vi "TJR_StateMachine.vi"() -> ()   [LabVIEW 2015]
uses:
  <vilib>/Utility/error.llb/DialogType.ctl
  <vilib>/DAQmx/read.llb/DAQmx Read (Analog 2D DBL NChan NSamp).vi
  <vilib>/DAQmx/configure/timing.llb/DAQmx Timing (Sample Clock).vi
  <vilib>/DAQmx/miscellaneous.llb/DAQmx Fill In Error Info.vi
  <vilib>/measure/maspectr.llb/Frequency Response Function (Mag-Phase) 1-1.vi
  <vilib>/express/express analysis/Spectral/Block/exnSpectralBlock spectral measurements RMS poly.vi
  <vilib>/express/express analysis/Spectral/Block/exnSpectralBlock spectral measurements RMS DDT.vi
  <vilib>/express/express analysis/Spectral/XNode/ExpressSpectralMeasurementsBlockNode.xnode
  <resource>/objmgr/daqmx.rc
  <vilib>/measure/NI_MAPro.lvlib
panel:
  in  "Tab Control":T1(tab)
  out "Measurement 8":dbl[](graph)
  out "Measurement 7":dbl[](graph)
  out "Measurement 6":dbl[](graph)
  out "Measurement 5":dbl[](graph)
  in  "Physical Channel 8":tag caption="Physical Channel"
  in  "Channel Name 8":string caption="Channel 8 Name"
  in  "Physical Channel 6":tag caption="Physical Channel"
  in  "Channel Name 6":string caption="Channel 6 Name"
  in  "Ch 8 On/Off":bool
  in  "Ch 6 On/Off":bool
  in  "Channel Type 8":u16(ring) caption="Channel Type" items=["Voltage", "Acceleration", "Current", "Other"]
  in  "Channel Type 7":u16(ring) caption="Channel Type" items=["Voltage", "Acceleration", "Current", "Other"]
  in  "Scale Factor 8":dbl[unit]=1.0
  in  "Scale Factor 6":dbl[unit]=1.0
  out "Ch 6 LED":bool
  out "Ch 8 LED":bool
  in  "Physical Channel 1":tag caption="Physical Channel"
  in  "Channel Name 1":string caption="Channel 1 Name"
  in  "Physical Channel 2":tag caption="Physical Channel"
  in  "Channel Name 2":string caption="Channel 2 Name"
  in  "Physical Channel 3":tag caption="Physical Channel"
  in  "Channel Name 3":string caption="Channel 3 Name"
  in  "Physical Channel 4":tag caption="Physical Channel"
  in  "Channel Name 4":string caption="Channel 4 Name"
  in  "Ch 1 On/Off":bool
  in  "Ch 2 On/Off":bool
  in  "Ch 3 On/Off":bool
  in  "Ch 4 On/Off":bool
  in  "Channel Type 1":u16(ring) caption="Channel Type" items=["Voltage", "Acceleration", "Current", "Other"]
  in  "Channel Type 3":u16(ring) caption="Channel Type" items=["Voltage", "Acceleration", "Current", "Other"]
  in  "Channel Type 4":u16(ring) caption="Channel Type" items=["Voltage", "Acceleration", "Current", "Other"]
  in  "Channel Type 2":u16(ring) caption="Channel Type" items=["Voltage", "Acceleration", "Current", "Other"]
  in  "Scale Factor 1":dbl[unit]=1.0 caption="mV/g"
  in  "Scale Factor 2":dbl[unit]=1.0 caption="mV/g"
  in  "Scale Factor 3":dbl[unit]=1.0 caption="mV/g"
  in  "Scale Factor 4":dbl[unit]=1.0
  in  "Rate":dbl=10.0 caption="Sampling Rate (Hz)" min=0.0 format="%0.2f"
  in  "Refresh Rate":dbl=5.0 caption="Refresh Rate (Hz)" min=1.0 max=20.0 step=1.0
  out "Measurement":dbl[](graph) caption="Input"
  out "Measurement 2":dbl[](graph) caption="A1"
  out "Measurement 3":dbl[](graph) caption="A2"
  out "Measurement 4":dbl[](graph) caption="A3"
  in  "Stop Acquisition":bool caption="stop"
  in  "Graph Time":dbl=10.0 caption="Graph Display Time (sec)" min=1.0 step=1.0
  out "Sampling Freq":dbl caption="Actual Sample Rate (Hz)"
  in  "Start Acquisition":bool
  in  "Exit":bool
  out "Ch 4 LED":bool
  out "Ch 3 LED":bool
  out "Ch 2 LED":bool
  out "Ch 1 LED":bool
  out "Ch 5 LED":bool
  in  "Scale Factor 5":dbl[unit]=1.0
  in  "Channel Type 6":u16(ring) caption="Channel Type" items=["Voltage", "Acceleration", "Current", "Other"]
  in  "Ch 5 On/Off":bool
  in  "Channel Name 5":string caption="Channel 5 Name"
  in  "Physical Channel 5":tag caption="Physical Channel"
  out "Ch 7 LED":bool
  in  "Scale Factor 7":dbl[unit]=1.0
  in  "Channel Type 5":u16(ring) caption="Channel Type" items=["Voltage", "Acceleration", "Current", "Other"]
  in  "Ch 7 On/Off":bool
  in  "Channel Name 7":string caption="Channel 7 Name"
  in  "Physical Channel 7":tag caption="Physical Channel"
  in  "Input Signal Measurement Channel":string(combo)
  out "A/O LED":bool
  out "Resulting Frequency":dbl=1000.0 format="%.4f"
  in  "Cycles per Buffer":i32=5 min=0 step=1
  in  "Waveform Type":T2(ring)
  in  "Amplitude":dbl=1.0 format="%.4f"
  in  "Analog Ouput On/Off":bool
  in  "Channel Name":string
  in  "Physical Channel":tag
  in  "Desired Frequency":dbl=100.0 min=0.0 format="%.4f"
  out "FFT Magnitude":dynamicdata(graph)
  out "FFT Phase":dynamicdata(graph)
  out "FRF Magnitude":cluster{"f0":dbl, "df":dbl, "magnitude":dbl[]}[](graph)
  out "FRF Phase":cluster{"f0":dbl, "df":dbl, "phase":dbl[]}[](graph)
  out "FRF Coherence":cluster{"f0":dbl, "df":dbl, "coherence":dbl[]}[](graph)
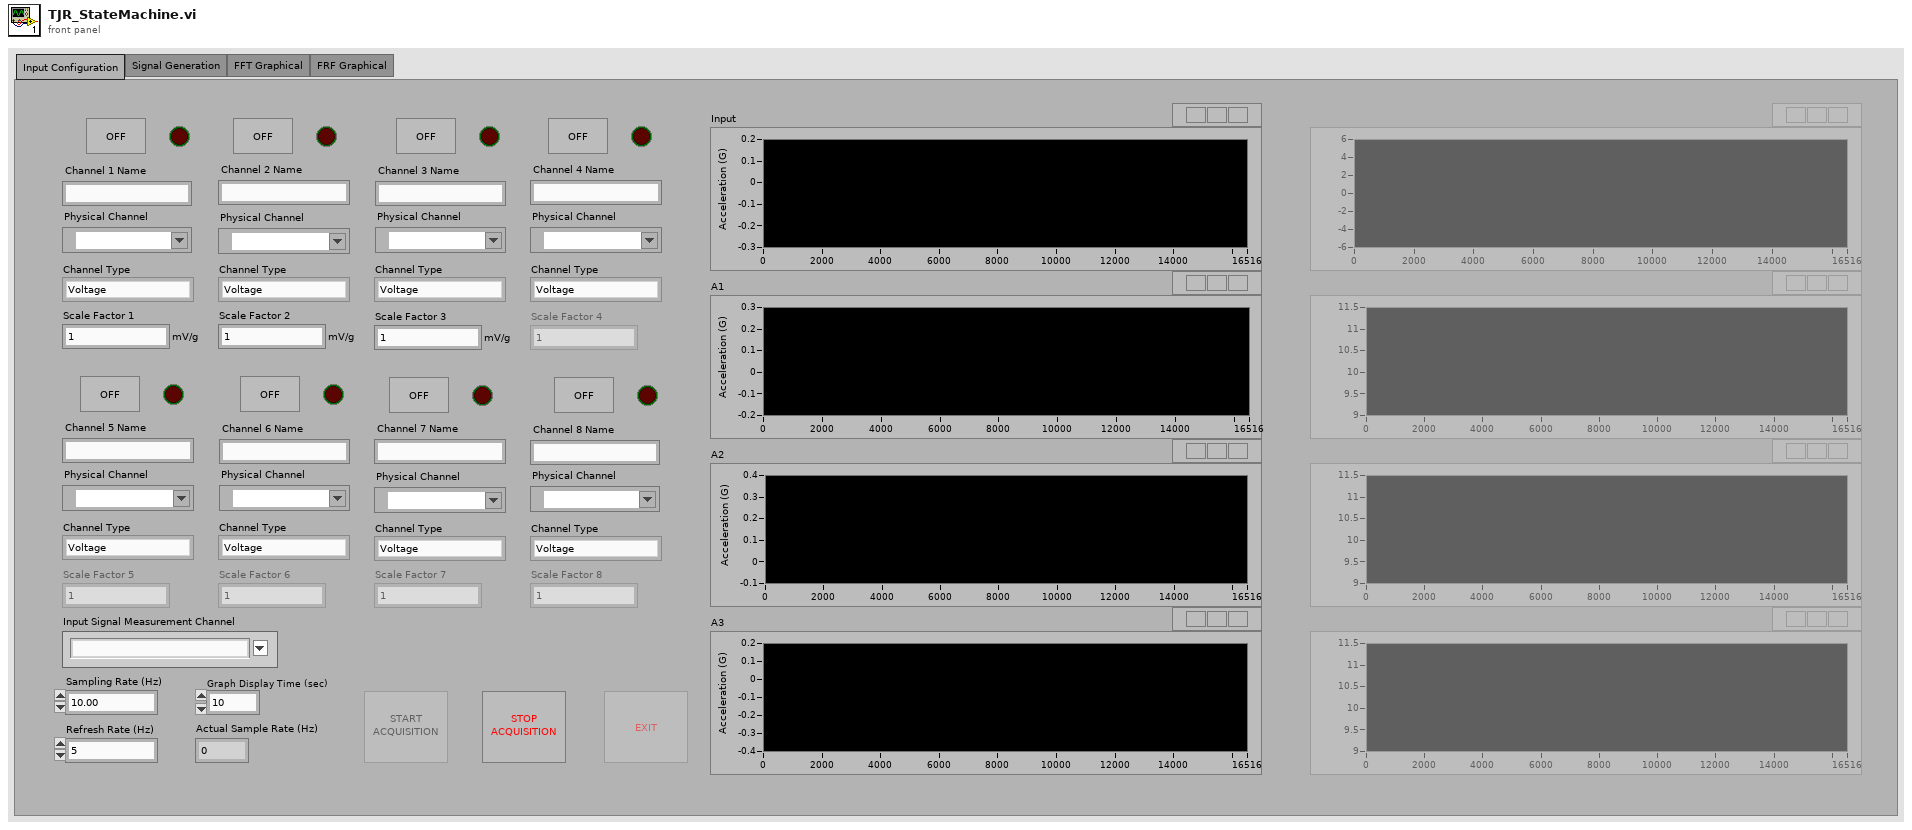
[diagram p1: front panel]
types:
  T1 = enum32{"Input Configuration", "Signal Generation", "FFT Graphical", "FRF Graphical"}
  T2 = enum16{"Sine Wave", "Triangle Wave", "Square Wave", "Sawtooth Wave"}
  T3 = cluster{"averaging mode":u16, "weighting mode":u16, "number of averages":u32}
  T4 = cluster{"dB On (F)":bool, "unwrap phase (F)":bool, "convert to degree (F)":bool}
  T5 = cluster{"Ch 1 On/Off":bool, "Ch 2 On/Off":bool, "Ch 3 On/Off":bool, "Ch 4 On/Off":bool, "Ch 5 On/Off":bool, "Ch 6 On/Off":bool, "Ch 7 On/Off":bool, "Ch 8 On/Off ":bool}
  T6 = cluster{"Physical Channel 1":tag, "Physical Channel 2":tag, "Physical Channel 3":tag, "Physical Channel 4":tag, "Physical Channel 5":tag, "Physical Channel 6":tag, "Physical Channel 7":tag, "Physical Channel 8":tag}
  T7 = cluster{"Minimum Value (V) 1":dbl, "Minimum Value (V) 2":dbl, "Minimum Value (V) 3":dbl, "Minimum Value (V) 4":dbl, "Minimum Value (V) 5":dbl, "Minimum Value (V) 6":dbl, "Minimum Value (V) 7":dbl, "Minimum Value (V) 8":dbl}
  T8 = cluster{"Scale Factor 8":dbl[unit], "Scale Factor 7":dbl[unit], "Scale Factor 6":dbl[unit], "Scale Factor 5":dbl[unit], "Scale Factor 4":dbl[unit], "Scale Factor 3":dbl[unit], "Scale Factor 2":dbl[unit], "Scale Factor 1":dbl[unit]}
  T9 = cluster{"Maximum Value (V) 1":dbl, "Maximum Value (V) 2":dbl, "Maximum Value (V) 3":dbl, "Maximum Value (V) 4":dbl, "Maximum Value (V) 5":dbl, "Maximum Value (V) 6":dbl, "Maximum Value (V) 7":dbl, "Maximum Value (V) 8":dbl}
  T10 = cluster{"Channel Name 1":string, "Channel Name 2":string, "Channel Name 3":string, "Channel Name 4":string, "Channel Name 5":string, "Channel Name 6":string, "Channel Name 7":string, "Channel Name 8":string}
  T11 = cluster{"Channel Type 1":u16, "Channel Type 2":u16, "Channel Type 3":u16, "Channel Type 4":u16, "Channel Type 5":u16, "Channel Type 6":u16, "Channel Type 7":u16, "Channel Type 8":u16}
  T12 = cluster{"Measurement":refnum<vi>, "Measurement 2":refnum<vi>, "Measurement 3":refnum<vi>, "Measurement 4":refnum<vi>, "Measurement 5":refnum<vi>, "Measurement 6":refnum<vi>, "Measurement 7":refnum<vi>, "Measurement 8":refnum<vi>}
  T13 = cluster{cluster{"Measurement":refnum<vi>, "Measurement 2":refnum<vi>, "Measurement 3":refnum<vi>, "Measurement 4":refnum<vi>, "Measurement 5":refnum<vi>, "Measurement 6":refnum<vi>, "Measurement 7":refnum<vi>, "Measurement 8":refnum<vi>}, cluster{"Ch 1 On/Off":bool, "Ch 2 On/Off":bool, "Ch 3 On/Off":bool, "Ch 4 On/Off":bool, "Ch 5 On/Off":bool, "Ch 6 On/Off":bool, "Ch 7 On/Off":bool, "Ch 8 On/Off ":bool}, cluster{"Channel Name 1":string, "Channel Name 2":string, "Channel Name 3":string, "Channel Name 4":string, "Channel Name 5":string, "Channel Name 6":string, "Channel Name 7":string, "Channel Name 8":string}, cluster{"Physical Channel 1":tag, "Physical Channel 2":tag, "Physical Channel 3":tag, "Physical Channel 4":tag, "Physical Channel 5":tag, "Physical Channel 6":tag, "Physical Channel 7":tag, "Physical Channel 8":tag}, cluster{"Maximum Value (V) 1":dbl, "Maximum Value (V) 2":dbl, "Maximum Value (V) 3":dbl, "Maximum Value (V) 4":dbl, "Maximum Value (V) 5":dbl, "Maximum Value (V) 6":dbl, "Maximum Value (V) 7":dbl, "Maximum Value (V) 8":dbl}, cluster{"Minimum Value (V) 1":dbl, "Minimum Value (V) 2":dbl, "Minimum Value (V) 3":dbl, "Minimum Value (V) 4":dbl, "Minimum Value (V) 5":dbl, "Minimum Value (V) 6":dbl, "Minimum Value (V) 7":dbl, "Minimum Value (V) 8":dbl}, cluster{"Channel Type 1":u16, "Channel Type 2":u16, "Channel Type 3":u16, "Channel Type 4":u16, "Channel Type 5":u16, "Channel Type 6":u16, "Channel Type 7":u16, "Channel Type 8":u16}, cluster{"Scale Factor 8":dbl[unit], "Scale Factor 7":dbl[unit], "Scale Factor 6":dbl[unit], "Scale Factor 5":dbl[unit], "Scale Factor 4":dbl[unit], "Scale Factor 3":dbl[unit], "Scale Factor 2":dbl[unit], "Scale Factor 1":dbl[unit]}}
  T14 = typedef "DialogType.ctl" = u16
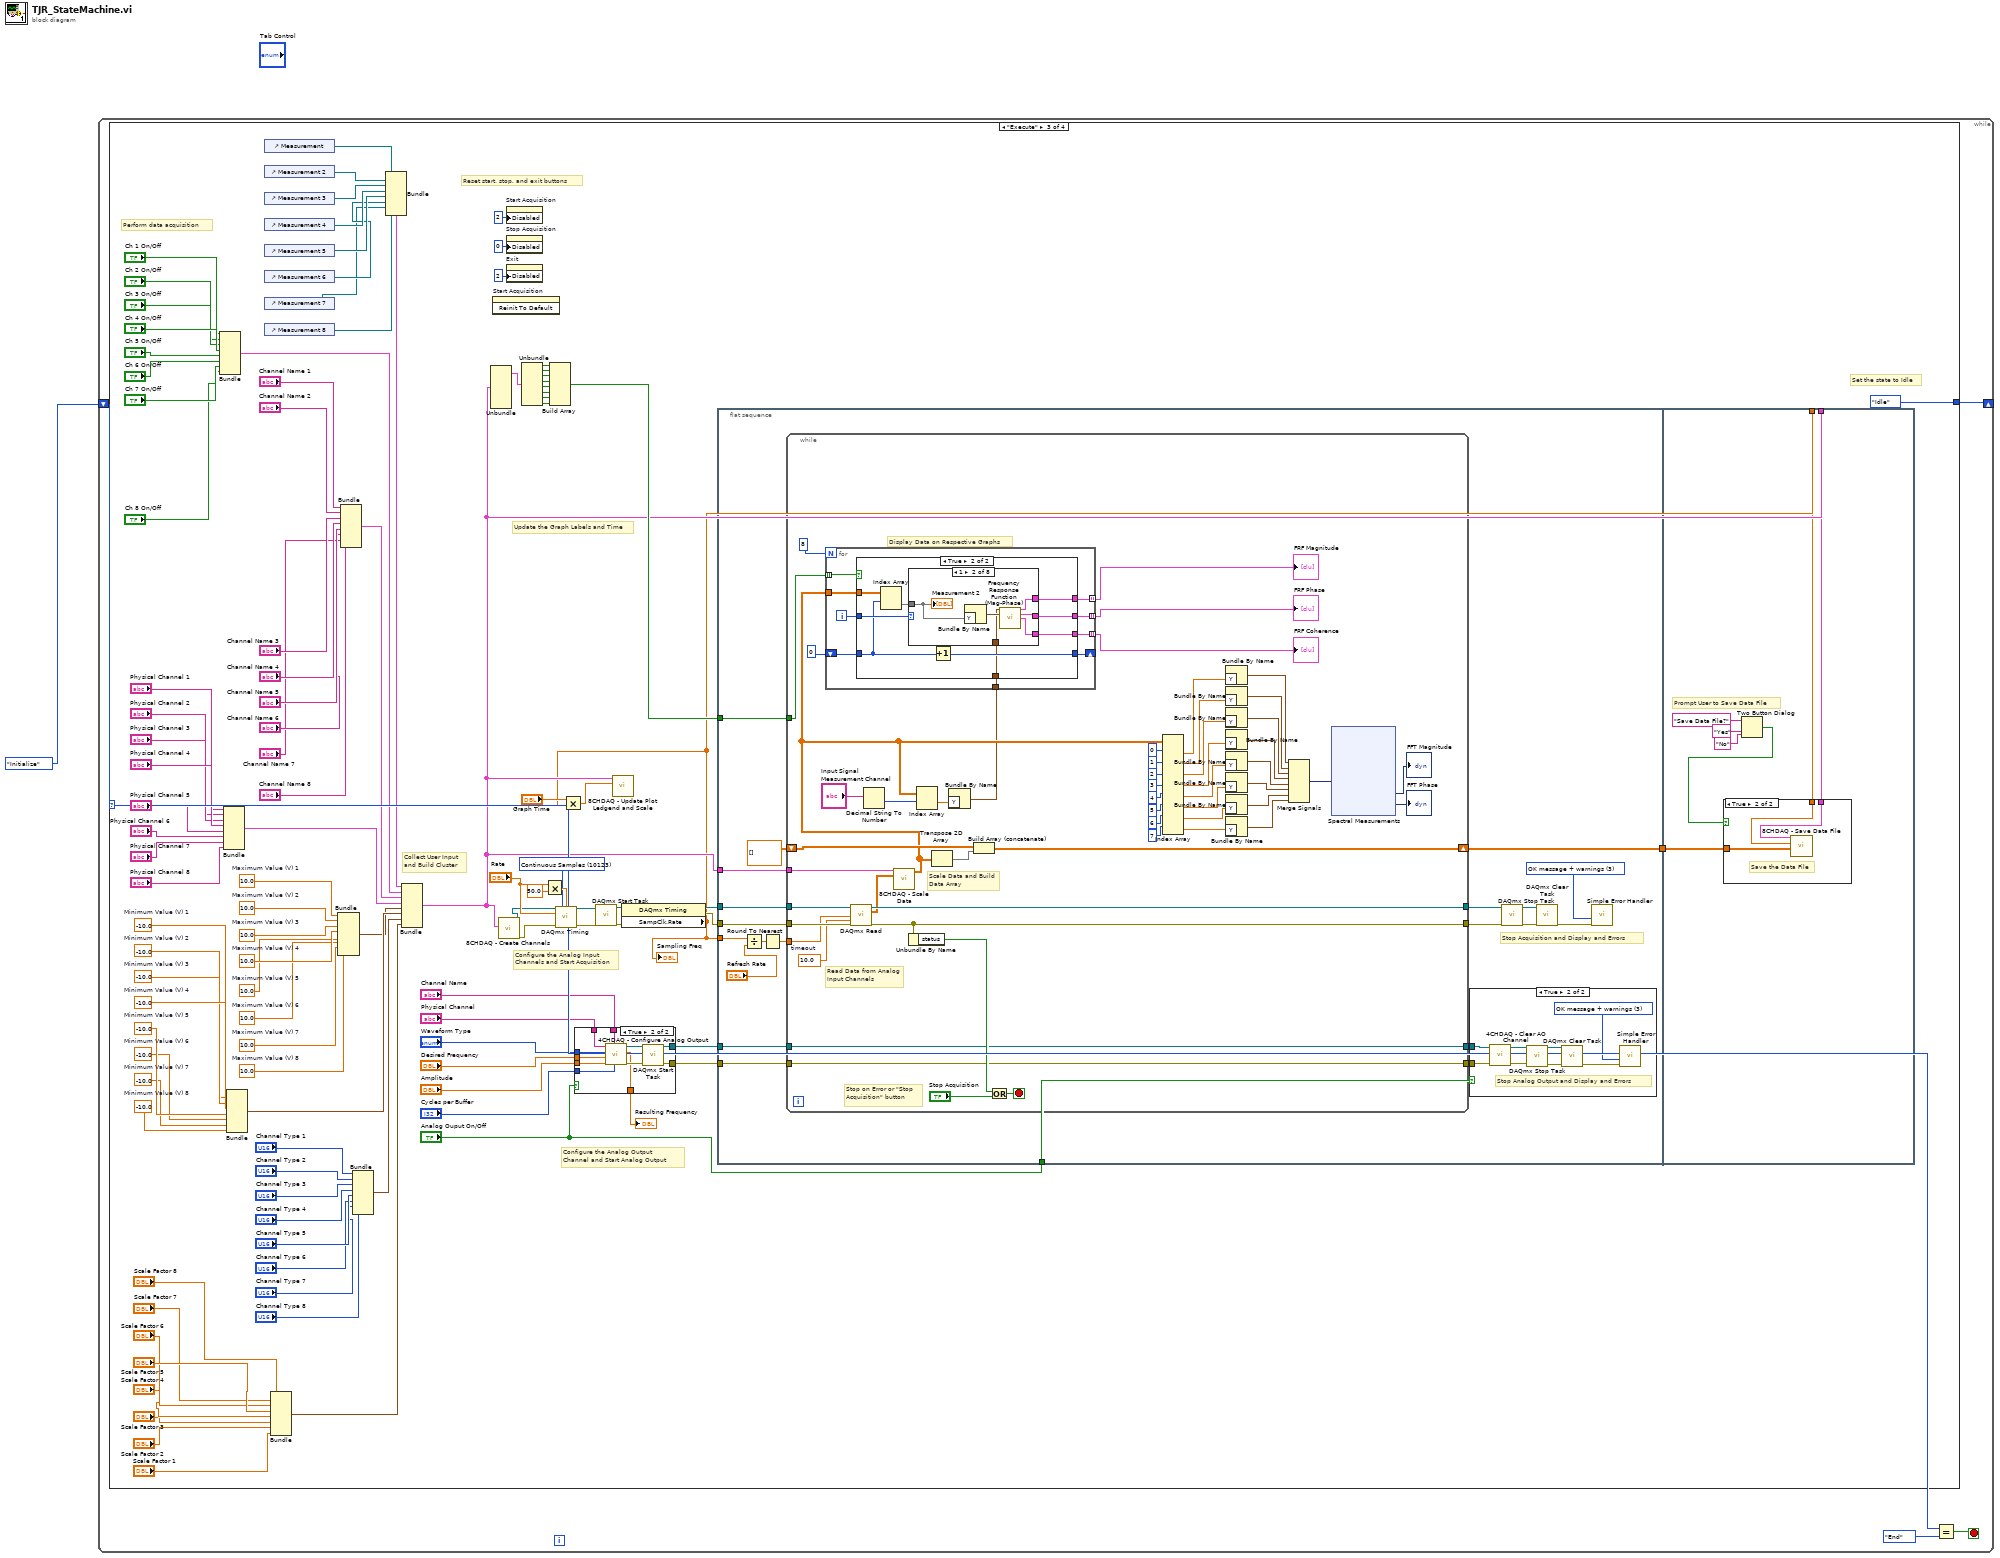
[diagram p0: block diagram]
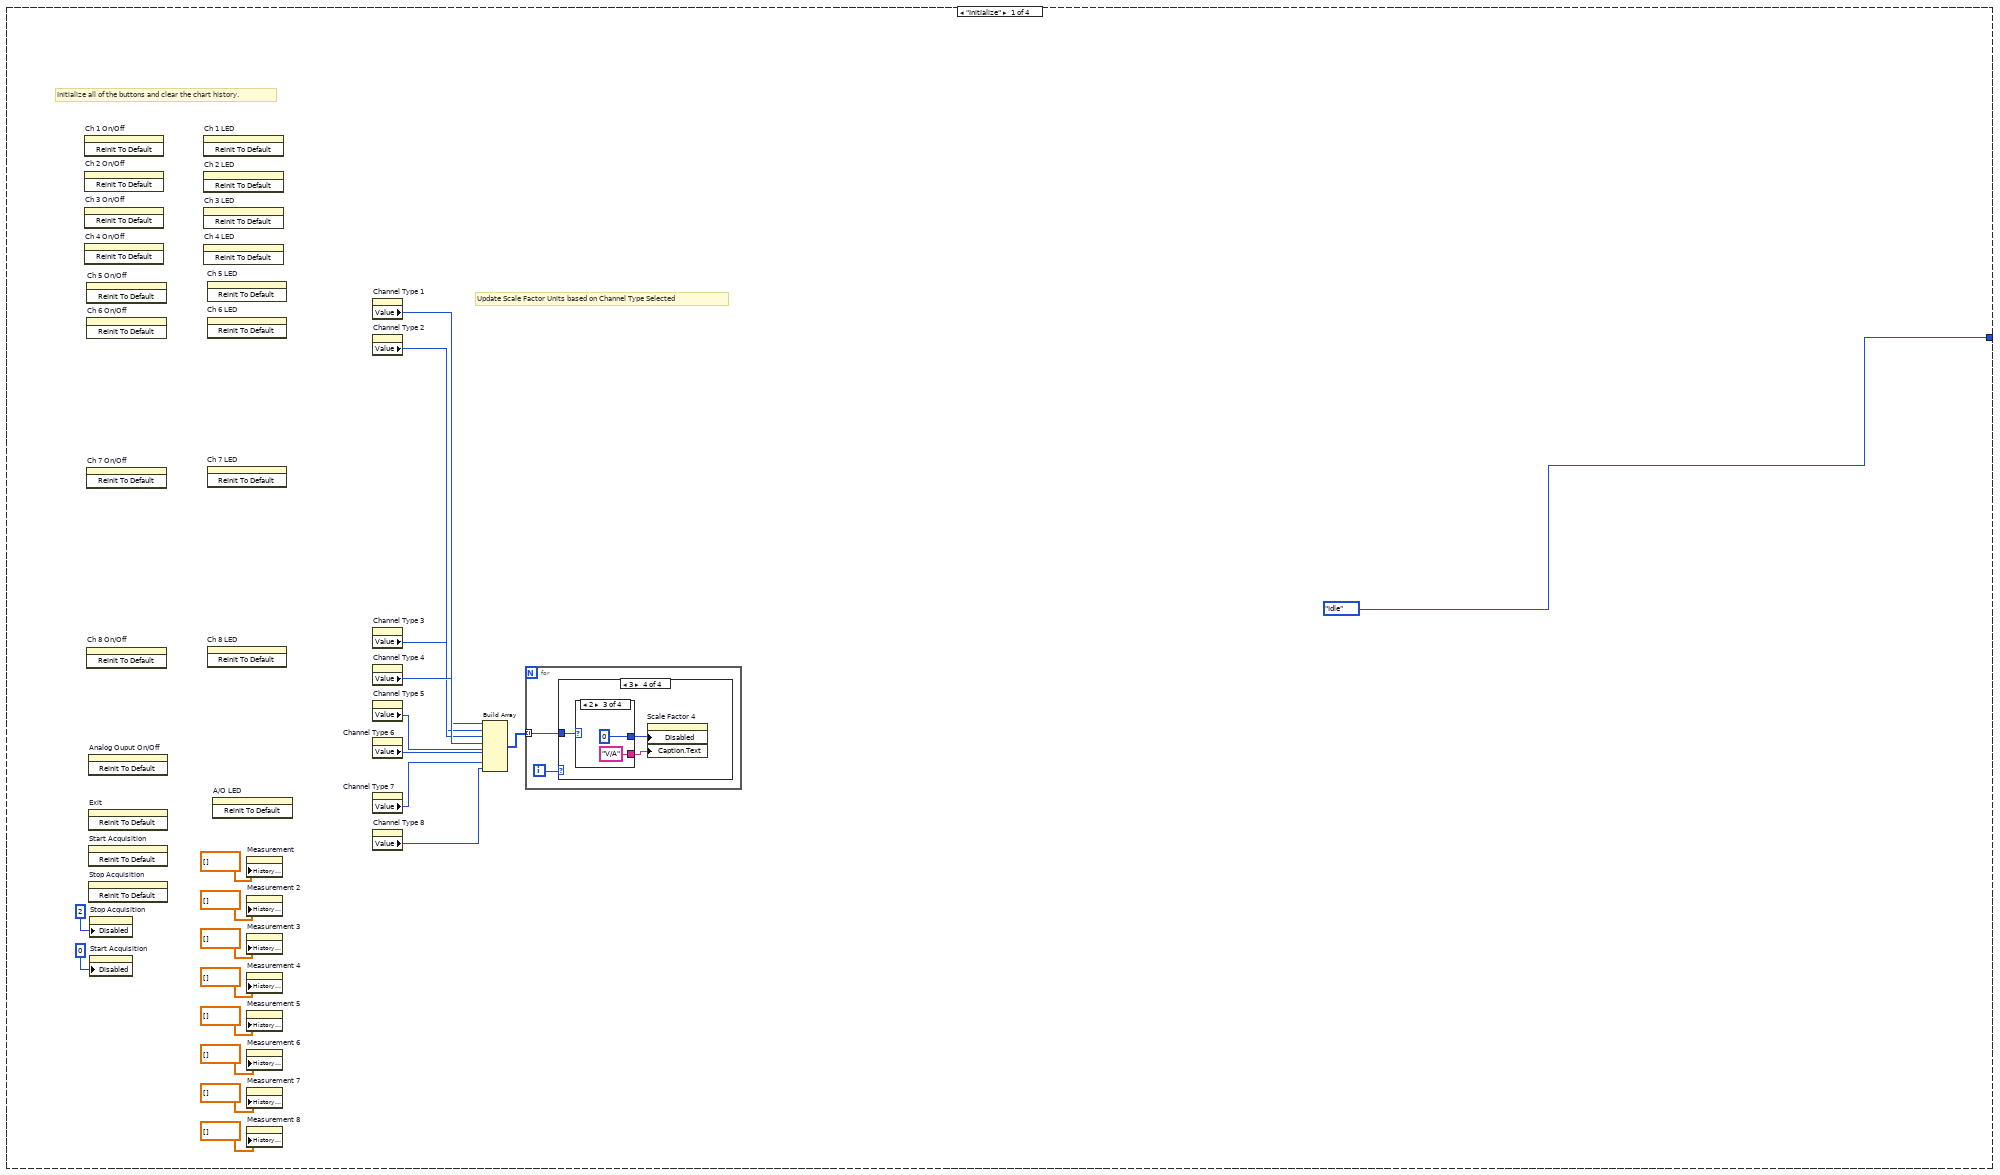
[diagram p2: hidden frame]
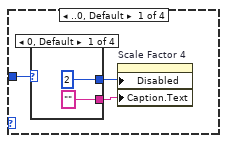
[diagram p3: hidden frame]
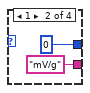
[diagram p4: hidden frame]
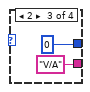
[diagram p5: hidden frame]
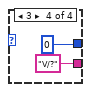
[diagram p6: hidden frame]
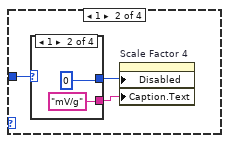
[diagram p7: hidden frame]
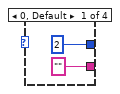
[diagram p8: hidden frame]
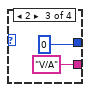
[diagram p9: hidden frame]
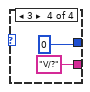
[diagram p10: hidden frame]
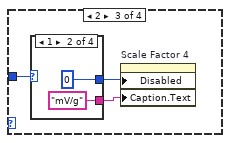
[diagram p11: hidden frame]
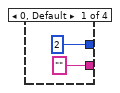
[diagram p12: hidden frame]
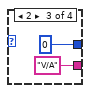
[diagram p13: hidden frame]
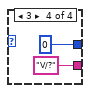
[diagram p14: hidden frame]
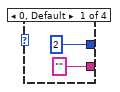
[diagram p15: hidden frame]
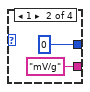
[diagram p16: hidden frame]
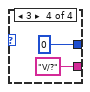
[diagram p17: hidden frame]
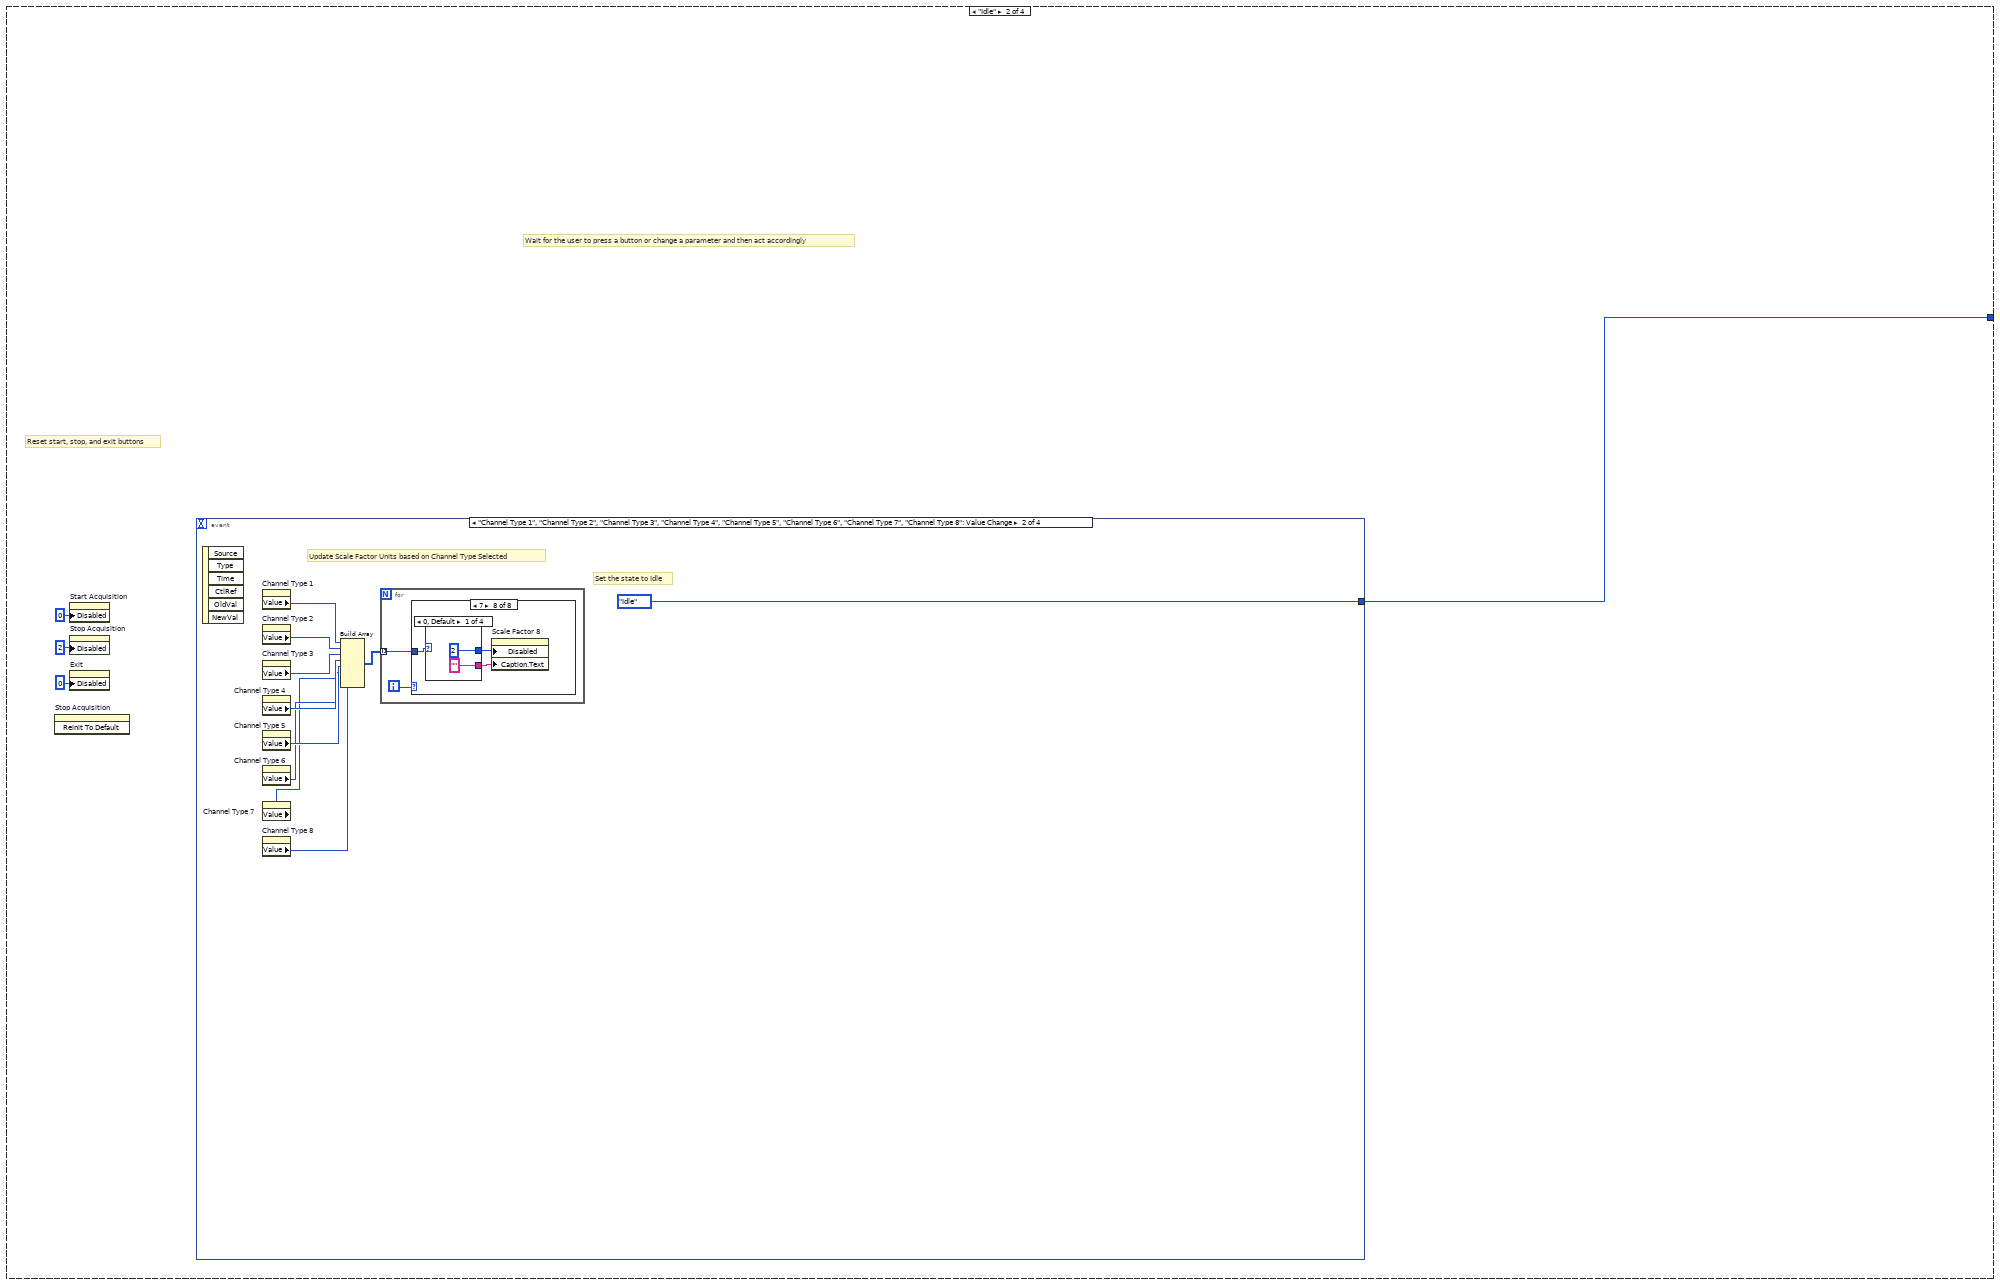
[diagram p18: hidden frame]
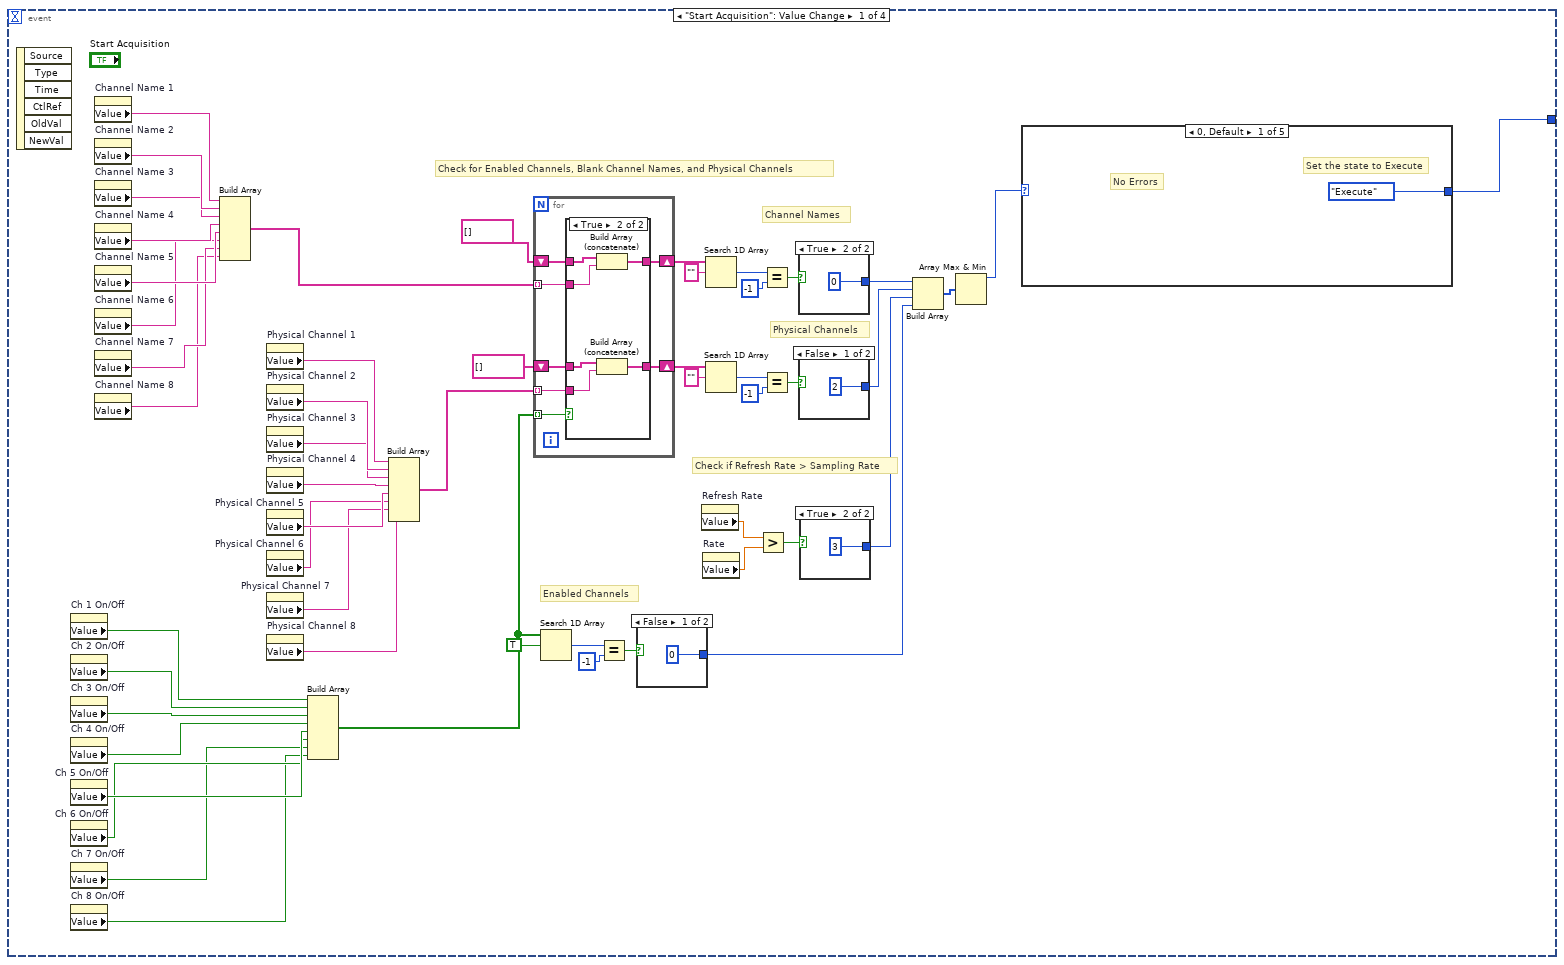
[diagram p19: hidden frame]
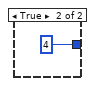
[diagram p20: hidden frame]
diagram:
  n1 = while {
    shift-right: [w2] -> _
    shift-left: enum16{"Initialize", "Idle", "Execute", "End"}."Initialize" -> [w3]
    stop <- w5 stop-if-true
    n2 = case shown="\"Execute\"" w3 {
      tunnel: [enum16{"Initialize", "Idle", "Execute", "End"}."Idle" w72 enum16{"Initialize", "Idle", "Execute", "End"}."Idle" enum16{"Initialize", "Idle", "Execute", "End"}."Idle"] -> w2
      frame "Initialize" {
        # "Update Scale Factor Units based on Channel Type Selected"
        # "Initialize all of the buttons and clear the chart history."
        n3 = invoke on="Ch 1 On/Off" class="Bool (strict)" method="Reinit To Default"() -> ()  [unwired: 3 in, 3 out]
        n4 = invoke on="Ch 2 On/Off" class="Bool (strict)" method="Reinit To Default"() -> ()  [unwired: 3 in, 3 out]
        n5 = invoke on="Ch 3 On/Off" class="Bool (strict)" method="Reinit To Default"() -> ()  [unwired: 3 in, 3 out]
        n6 = invoke on="Ch 4 On/Off" class="Bool (strict)" method="Reinit To Default"() -> ()  [unwired: 3 in, 3 out]
        n7 = invoke on="Ch 5 On/Off" class="Bool (strict)" method="Reinit To Default"() -> ()  [unwired: 3 in, 3 out]
        n8 = invoke on="Ch 6 On/Off" class="Bool (strict)" method="Reinit To Default"() -> ()  [unwired: 3 in, 3 out]
        n9 = invoke on="Ch 7 On/Off" class="Bool (strict)" method="Reinit To Default"() -> ()  [unwired: 3 in, 3 out]
        n10 = invoke on="Ch 8 On/Off" class="Bool (strict)" method="Reinit To Default"() -> ()  [unwired: 3 in, 3 out]
        n11 = invoke on="Analog Ouput On/Off" class="Bool (strict)" method="Reinit To Default"() -> ()  [unwired: 3 in, 3 out]
        n12 = invoke on="Exit" class="Bool (strict)" method="Reinit To Default"() -> ()  [unwired: 3 in, 3 out]
        n13 = invoke on="Start Acquisition" class="Bool (strict)" method="Reinit To Default"() -> ()  [unwired: 3 in, 3 out]
        n14 = invoke on="Stop Acquisition" class="Bool (strict)" method="Reinit To Default"() -> ()  [unwired: 3 in, 3 out]
        n15 = property on="Stop Acquisition" class="Bool (strict)"("Disabled"=u8 2) -> ()  [unwired: 2 in, 2 out]
        n16 = property on="Start Acquisition" class="Bool (strict)"("Disabled"=u8 0) -> ()  [unwired: 2 in, 2 out]
        n17 = invoke on="Ch 1 LED" class="Bool (strict)" method="Reinit To Default"() -> ()  [unwired: 3 in, 3 out]
        n18 = invoke on="Ch 2 LED" class="Bool (strict)" method="Reinit To Default"() -> ()  [unwired: 3 in, 3 out]
        n19 = invoke on="Ch 3 LED" class="Bool (strict)" method="Reinit To Default"() -> ()  [unwired: 3 in, 3 out]
        n20 = invoke on="Ch 4 LED" class="Bool (strict)" method="Reinit To Default"() -> ()  [unwired: 3 in, 3 out]
        n21 = invoke on="Ch 5 LED" class="Bool (strict)" method="Reinit To Default"() -> ()  [unwired: 3 in, 3 out]
        n22 = invoke on="Ch 6 LED" class="Bool (strict)" method="Reinit To Default"() -> ()  [unwired: 3 in, 3 out]
        n23 = invoke on="Ch 7 LED" class="Bool (strict)" method="Reinit To Default"() -> ()  [unwired: 3 in, 3 out]
        n24 = invoke on="Ch 8 LED" class="Bool (strict)" method="Reinit To Default"() -> ()  [unwired: 3 in, 3 out]
        n25 = invoke on="A/O LED" class="Bool (strict)" method="Reinit To Default"() -> ()  [unwired: 3 in, 3 out]
        n26 = property on="Measurement" class="WFChart (strict)"("History Data"=dbl[] []) -> ()  [unwired: 2 in, 2 out]
        n27 = property on="Measurement 2" class="WFChart (strict)"("History Data"=dbl[] []) -> ()  [unwired: 2 in, 2 out]
        n28 = property on="Measurement 3" class="WFChart (strict)"("History Data"=dbl[] []) -> ()  [unwired: 2 in, 2 out]
        n29 = property on="Measurement 4" class="WFChart (strict)"("History Data"=dbl[] []) -> ()  [unwired: 2 in, 2 out]
        n30 = property on="Measurement 5" class="WFChart (strict)"("History Data"=dbl[] []) -> ()  [unwired: 2 in, 2 out]
        n31 = property on="Measurement 6" class="WFChart (strict)"("History Data"=dbl[] []) -> ()  [unwired: 2 in, 2 out]
        n32 = property on="Measurement 7" class="WFChart (strict)"("History Data"=dbl[] []) -> ()  [unwired: 2 in, 2 out]
        n33 = property on="Measurement 8" class="WFChart (strict)"("History Data"=dbl[] []) -> ()  [unwired: 2 in, 2 out]
        n34 = property on="Channel Type 1" class="Ring (strict)"() -> ("Value"=w22:u16)  [unwired: 2 in, 2 out]
        n35 = property on="Channel Type 2" class="Ring (strict)"() -> ("Value"=w23:u16)  [unwired: 2 in, 2 out]
        n36 = property on="Channel Type 3" class="Ring (strict)"() -> ("Value"=w24:u16)  [unwired: 2 in, 2 out]
        n37 = property on="Channel Type 4" class="Ring (strict)"() -> ("Value"=w25:u16)  [unwired: 2 in, 2 out]
        n38 = property on="Channel Type 5" class="Ring (strict)"() -> ("Value"=w9:u16)  [unwired: 2 in, 2 out]
        n39 = property on="Channel Type 6" class="Ring (strict)"() -> ("Value"=w8:u16)  [unwired: 2 in, 2 out]
        n40 = property on="Channel Type 7" class="Ring (strict)"() -> ("Value"=w7:u16)  [unwired: 2 in, 2 out]
        n41 = property on="Channel Type 8" class="Ring (strict)"() -> ("Value"=w6:u16)  [unwired: 2 in, 2 out]
        n42 = Build Array(w22, w23, w24, w25, w9, w8, w7, w6) -> (w21:u16[])
        n43 = for {
          tunnel: w21 -> [w27] mode=indexing
          i -> [w26]
          n44 = case shown="3" w26 {
            tunnel: w27 -> [w30 w41 w52 w63]
            frame ..0, Default {
              n45 = case shown="0, Default" w30 {
                tunnel: [2 0 0 0] -> w29
                tunnel: ["" ("Caption.Text") "mV/g" ("Caption.Text") "V/A" ("Caption.Text") "V/?" ("Caption.Text")] -> w28
                frame 0, Default {
                }
                frame 1 {
                }
                frame 2 {
                }
                frame 3 {
                }
              }
              n46 = property on="Scale Factor 4" class="DigNum (strict)"("Disabled"=w29, "Caption.Text"=w28) -> ()  [unwired: 2 in, 2 out]
            }
            frame 1 {
              n47 = case shown="1" w41 {
                tunnel: [2 0 0 0] -> w40
                tunnel: ["" ("Caption.Text") "mV/g" ("Caption.Text") "V/A" ("Caption.Text") "V/?" ("Caption.Text")] -> w39
                frame 0, Default {
                }
                frame 1 {
                }
                frame 2 {
                }
                frame 3 {
                }
              }
              n48 = property on="Scale Factor 4" class="DigNum (strict)"("Disabled"=w40, "Caption.Text"=w39) -> ()  [unwired: 2 in, 2 out]
            }
            frame 2 {
              n49 = case shown="1" w52 {
                tunnel: [2 0 0 0] -> w51
                tunnel: ["" ("Caption.Text") "mV/g" ("Caption.Text") "V/A" ("Caption.Text") "V/?" ("Caption.Text")] -> w50
                frame 0, Default {
                }
                frame 1 {
                }
                frame 2 {
                }
                frame 3 {
                }
              }
              n50 = property on="Scale Factor 4" class="DigNum (strict)"("Disabled"=w51, "Caption.Text"=w50) -> ()  [unwired: 2 in, 2 out]
            }
            frame 3 {
              n51 = case shown="2" w63 {
                tunnel: [2 0 0 0] -> w62
                tunnel: ["" ("Caption.Text") "mV/g" ("Caption.Text") "V/A" ("Caption.Text") "V/?" ("Caption.Text")] -> w61
                frame 0, Default {
                }
                frame 1 {
                }
                frame 2 {
                }
                frame 3 {
                }
              }
              n52 = property on="Scale Factor 4" class="DigNum (strict)"("Disabled"=w62, "Caption.Text"=w61) -> ()  [unwired: 2 in, 2 out]
            }
          }
        }
      }
      frame "Idle" {
        # "Wait for the user to press a button or change a parameter and then act accordingly"
        # "Reset start, stop, and exit buttons"
        n53 = invoke on="Stop Acquisition" class="Bool (strict)" method="Reinit To Default"() -> ()  [unwired: 3 in, 3 out]
        n54 = property on="Start Acquisition" class="Bool (strict)"("Disabled"=u8 0) -> ()  [unwired: 2 in, 2 out]
        n55 = property on="Stop Acquisition" class="Bool (strict)"("Disabled"=u8 2) -> ()  [unwired: 2 in, 2 out]
        n56 = property on="Exit" class="Bool (strict)"("Disabled"=u8 0) -> ()  [unwired: 2 in, 2 out]
        n57 = event shown="[1] \"Channel Type 1\", \"Channel Type 2\", \"Channel Type 3\", \"Channel Type 4\", \"Channel Type 5\", \"Channel Type 6\", \"Channel Type 7\", \"Channel Type 8\": Value Change" {
          selector: _ -> [_ _ _ _]
          dyn-events: _ -> [_ _ _ _]
          timeout: _ -> [_ _ _ _]
          tunnel: [w128 enum16{"Initialize", "Idle", "Execute", "End"}."Idle" enum16{"Initialize", "Idle", "Execute", "End"}."Idle" enum16{"Initialize", "Idle", "Execute", "End"}."End"] -> w72
          event "Start Acquisition": Value Change {
            # "Enabled Channels"
            # "Physical Channels"
            # "Channel Names"
            # "Check if Refresh Rate > Sampling Rate"
            # "Check for Enabled Channels, Blank Channel Names, and Physical Channels"
            n58 = event-data() -> ()  [unwired: 1 in, 6 out]
            n59 = property on="Ch 1 On/Off" class="Bool (strict)"() -> ("Value"=w122:bool)  [unwired: 2 in, 2 out]
            n60 = property on="Ch 2 On/Off" class="Bool (strict)"() -> ("Value"=w121:bool)  [unwired: 2 in, 2 out]
            n61 = property on="Ch 3 On/Off" class="Bool (strict)"() -> ("Value"=w120:bool)  [unwired: 2 in, 2 out]
            n62 = property on="Ch 4 On/Off" class="Bool (strict)"() -> ("Value"=w119:bool)  [unwired: 2 in, 2 out]
            n63 = property on="Ch 5 On/Off" class="Bool (strict)"() -> ("Value"=w87:bool)  [unwired: 2 in, 2 out]
            n64 = property on="Ch 6 On/Off" class="Bool (strict)"() -> ("Value"=w86:bool)  [unwired: 2 in, 2 out]
            n65 = property on="Ch 7 On/Off" class="Bool (strict)"() -> ("Value"=w85:bool)  [unwired: 2 in, 2 out]
            n66 = property on="Ch 8 On/Off" class="Bool (strict)"() -> ("Value"=w84:bool)  [unwired: 2 in, 2 out]
            n67 = property on="Channel Name 1" class="Str"() -> ("Value"=w127:string)  [unwired: 2 in, 2 out]
            n68 = property on="Channel Name 2" class="Str"() -> ("Value"=w126:string)  [unwired: 2 in, 2 out]
            n69 = property on="Channel Name 3" class="Str"() -> ("Value"=w125:string)  [unwired: 2 in, 2 out]
            n70 = property on="Channel Name 4" class="Str"() -> ("Value"=w124:string)  [unwired: 2 in, 2 out]
            n71 = property on="Channel Name 5" class="Str"() -> ("Value"=w79:string)  [unwired: 2 in, 2 out]
            n72 = property on="Channel Name 6" class="Str"() -> ("Value"=w78:string)  [unwired: 2 in, 2 out]
            n73 = property on="Channel Name 7" class="Str"() -> ("Value"=w77:string)  [unwired: 2 in, 2 out]
            n74 = property on="Channel Name 8" class="Str"() -> ("Value"=w76:string)  [unwired: 2 in, 2 out]
            n75 = Build Array(w127, w126, w125, w124, w79, w78, w77, w76) -> (w118:string[])
            n76 = property on="Physical Channel 1" class="DAQmxName"() -> ("Value"=w106:string)  [unwired: 2 in, 2 out]
            n77 = property on="Physical Channel 2" class="DAQmxName"() -> ("Value"=w105:string)  [unwired: 2 in, 2 out]
            n78 = property on="Physical Channel 3" class="DAQmxName"() -> ("Value"=w104:string)  [unwired: 2 in, 2 out]
            n79 = property on="Physical Channel 4" class="DAQmxName"() -> ("Value"=w103:string)  [unwired: 2 in, 2 out]
            n80 = property on="Physical Channel 5" class="DAQmxName"() -> ("Value"=w83:string)  [unwired: 2 in, 2 out]
            n81 = property on="Physical Channel 6" class="DAQmxName"() -> ("Value"=w82:string)  [unwired: 2 in, 2 out]
            n82 = property on="Physical Channel 7" class="DAQmxName"() -> ("Value"=w81:string)  [unwired: 2 in, 2 out]
            n83 = property on="Physical Channel 8" class="DAQmxName"() -> ("Value"=w80:string)  [unwired: 2 in, 2 out]
            n84 = Build Array(w122, w121, w120, w119, w87, w86, w85, w84) -> (w93:bool[])
            n85 = Build Array(w106, w105, w104, w103, w83, w82, w81, w80) -> (w102:string[])
            n86 = for {
              tunnel: w93 -> [w152] mode=indexing
              tunnel: w118 -> [w151] mode=indexing
              shift-right: [w150] -> w116
              shift-left: string[] [] -> [w149]
              tunnel: w102 -> [w148] mode=indexing
              shift-right: [w147] -> w96
              shift-left: string[] [] -> [w146]
              n87 = case shown="True" w152 {
                tunnel: w151 -> [_ w159]
                tunnel: [w154 w160] -> w150
                tunnel: w149 -> [w154 w158]
                tunnel: w148 -> [_ w157]
                tunnel: [w153 w156] -> w147
                tunnel: w146 -> [w153 w155]
                frame False {
                }
                frame True {
                  n88 = Build Array (concatenate)(w158, w159) -> (w160:string[])
                  n89 = Build Array (concatenate)(w155, w157) -> (w156:string[])
                }
              }
            }
            n90 = Search 1D Array(1D array=w93, element=TRUE) -> (index of element=w90:i32)  [unwired: 1 in]
            n91 = Equal?(x=w90, y=-1) -> (x = y?=w89:bool)
            n92 = case shown="False" w89 {
              tunnel: [0 ("index of element") 4 ("index of element")] -> w88
              frame False {
              }
              frame True {
              }
            }
            n93 = property on="Refresh Rate" class="DigNum (strict)"() -> ("Value"=w113:dbl[unit])  [unwired: 2 in, 2 out]
            n94 = property on="Rate" class="DigNum (strict)"() -> ("Value"=w112:dbl[unit])  [unwired: 2 in, 2 out]
            n95 = Search 1D Array(1D array=w116, element="") -> (index of element=w114:i32)  [unwired: 1 in]
            n96 = Search 1D Array(1D array=w96, element="") -> (index of element=w99:i32)  [unwired: 1 in]
            n97 = Greater?(x=w113, y=w112) -> (0:w111:bool)
            n98 = Equal?(x=w114, y=-1) -> (x = y?=w110:bool)
            n99 = Equal?(x=w99, y=-1) -> (x = y?=w100:bool)
            n100 = case shown="True" w110 {
              tunnel: [1 ("index of element") 0 ("index of element")] -> w109
              frame False {
              }
              frame True {
              }
            }
            n101 = case shown="False" w100 {
              tunnel: [2 ("index of element") 0 ("index of element")] -> w94
              frame False {
              }
              frame True {
              }
            }
            n102 = case shown="True" w111 {
              tunnel: [0 ("index of element") 3 ("index of element")] -> w95
              frame False {
              }
              frame True {
              }
            }
            n103 = Build Array(w109, w94, w95, w88) -> (w108:i32[])
            n104 = Array Max & Min(array=w108) -> (max value=w107:i32)  [unwired: 3 out]
            n105 = case shown="0, Default" w107 {
              tunnel: [enum16{"Initialize", "Idle", "Execute", "End"}."Execute" enum16{"Initialize", "Idle", "Execute", "End"}."Idle" enum16{"Initialize", "Idle", "Execute", "End"}."Idle" enum16{"Initialize", "Idle", "Execute", "End"}."Idle" enum16{"Initialize", "Idle", "Execute", "End"}."Idle"] -> w128
              frame 0, Default {
                # "No Errors"
                # "Set the state to Execute"
              }
              frame 1 {
                # "Display Error Message to User"
                # "Set the State to Idle"
                n106 = invoke on="Start Acquisition" class="Bool (strict)" method="Reinit To Default"() -> ()  [unwired: 3 in, 3 out]
                n107 = One Button Dialog(message="One or more enabled channels have a blank Channel Name.\nPlease enter a Channel Name for these channels.") -> ()  [unwired: 1 in, 1 out]
              }
              frame 2 {
                # "Display Error Message to User"
                # "Set the State to Idle"
                n108 = invoke on="Start Acquisition" class="Bool (strict)" method="Reinit To Default"() -> ()  [unwired: 3 in, 3 out]
                n109 = One Button Dialog(message="One or more enabled channels have blank Physical Channels.\nPlease select Physical Channels for these channels.") -> ()  [unwired: 1 in, 1 out]
              }
              frame 3 {
                # "Display Error Message to User"
                # "Set the State to Idle"
                n110 = invoke on="Start Acquisition" class="Bool (strict)" method="Reinit To Default"() -> ()  [unwired: 3 in, 3 out]
                n111 = One Button Dialog(message="The Refresh Rate is set higher than the Sampling Frequency.\nPlease reduce the Refresh Rate below the Sampling Frequency.") -> ()  [unwired: 1 in, 1 out]
              }
              frame 4 {
                # "Display Error Message to User"
                # "Set the State to Idle"
                n112 = invoke on="Start Acquisition" class="Bool (strict)" method="Reinit To Default"() -> ()  [unwired: 3 in, 3 out]
                n113 = One Button Dialog(message="There are no Input Channels enabled.\nPlease enable at least one Input Channel.") -> ()  [unwired: 1 in, 1 out]
              }
            }
          }
          event "Channel Type 1", "Channel Type 2", "Channel Type 3", "Channel Type 4", "Channel Type 5", "Channel Type 6", "Channel Type 7", "Channel Type 8": Value Change {
            # "Set the state to Idle"
            # "Update Scale Factor Units based on Channel Type Selected"
            n114 = event-data() -> ()  [unwired: 1 in, 6 out]
            n115 = property on="Channel Type 1" class="Ring (strict)"() -> ("Value"=w168:u16)  [unwired: 2 in, 2 out]
            n116 = property on="Channel Type 2" class="Ring (strict)"() -> ("Value"=w167:u16)  [unwired: 2 in, 2 out]
            n117 = property on="Channel Type 3" class="Ring (strict)"() -> ("Value"=w166:u16)  [unwired: 2 in, 2 out]
            n118 = property on="Channel Type 4" class="Ring (strict)"() -> ("Value"=w165:u16)  [unwired: 2 in, 2 out]
            n119 = property on="Channel Type 5" class="Ring (strict)"() -> ("Value"=w164:u16)  [unwired: 2 in, 2 out]
            n120 = property on="Channel Type 6" class="Ring (strict)"() -> ("Value"=w163:u16)  [unwired: 2 in, 2 out]
            n121 = property on="Channel Type 7" class="Ring (strict)"() -> ("Value"=w162:u16)  [unwired: 2 in, 2 out]
            n122 = property on="Channel Type 8" class="Ring (strict)"() -> ("Value"=w161:u16)  [unwired: 2 in, 2 out]
            n123 = Build Array(w168, w167, w166, w165, w164, w163, w162, w161) -> (w169:u16[])
            n124 = for {
              tunnel: w169 -> [w172] mode=indexing
              i -> [w171]
              n125 = case shown="7" w171 {
                tunnel: w172 -> [w175 w186 w197 w208 w217 w228 w239 w250]
                frame ..0, Default {
                  n126 = case shown="0, Default" w175 {
                    tunnel: [2 0 0 0] -> w174
                    tunnel: ["" ("Caption.Text") "mV/g" ("Caption.Text") "V/A" ("Caption.Text") "V/?" ("Caption.Text")] -> w173
                    frame 0, Default {
                    }
                    frame 1 {
                    }
                    frame 2 {
                    }
                    frame 3 {
                    }
                  }
                  n127 = property on="Scale Factor 1" class="DigNum (strict)"("Disabled"=w174, "Caption.Text"=w173) -> ()  [unwired: 2 in, 2 out]
                }
                frame 1 {
                  n128 = case shown="1" w186 {
                    tunnel: [2 0 0 0] -> w185
                    tunnel: ["" ("Caption.Text") "mV/g" ("Caption.Text") "V/A" ("Caption.Text") "V/?" ("Caption.Text")] -> w184
                    frame 0, Default {
                    }
                    frame 1 {
                    }
                    frame 2 {
                    }
                    frame 3 {
                    }
                  }
                  n129 = property on="Scale Factor 2" class="DigNum (strict)"("Disabled"=w185, "Caption.Text"=w184) -> ()  [unwired: 2 in, 2 out]
                }
                frame 2 {
                  n130 = case shown="1" w197 {
                    tunnel: [2 0 0 0] -> w196
                    tunnel: ["" ("Caption.Text") "mV/g" ("Caption.Text") "V/A" ("Caption.Text") "V/?" ("Caption.Text")] -> w195
                    frame 0, Default {
                    }
                    frame 1 {
                    }
                    frame 2 {
                    }
                    frame 3 {
                    }
                  }
                  n131 = property on="Scale Factor 3" class="DigNum (strict)"("Disabled"=w196, "Caption.Text"=w195) -> ()  [unwired: 2 in, 2 out]
                }
                frame 3 {
                  n132 = case shown="1" w208 {
                    tunnel: [2 0 0 0] -> w207
                    tunnel: ["" ("Caption.Text") "mV/g" ("Caption.Text") "V/A" ("Caption.Text") "V/?" ("Caption.Text")] -> w206
                    frame 0, Default {
                    }
                    frame 1 {
                    }
                    frame 2 {
                    }
                    frame 3 {
                    }
                  }
                  n133 = property on="Scale Factor 4" class="DigNum (strict)"("Disabled"=w207, "Caption.Text"=w206) -> ()  [unwired: 2 in, 2 out]
                }
                frame 4 {
                  n134 = case shown="0, Default" w217 {
                    tunnel: [2 0 0 0] -> w219
                    tunnel: ["" ("Caption.Text") "mV/g" ("Caption.Text") "V/A" ("Caption.Text") "V/?" ("Caption.Text")] -> w218
                    frame 0, Default {
                    }
                    frame 1 {
                    }
                    frame 2 {
                    }
                    frame 3 {
                    }
                  }
                  n135 = property on="Scale Factor 5" class="DigNum (strict)"("Disabled"=w219, "Caption.Text"=w218) -> ()  [unwired: 2 in, 2 out]
                }
                frame 5 {
                  n136 = case shown="0, Default" w228 {
                    tunnel: [2 0 0 0] -> w229
                    tunnel: ["" ("Caption.Text") "mV/g" ("Caption.Text") "V/A" ("Caption.Text") "V/?" ("Caption.Text")] -> w230
                    frame 0, Default {
                    }
                    frame 1 {
                    }
                    frame 2 {
                    }
                    frame 3 {
                    }
                  }
                  n137 = property on="Scale Factor 6" class="DigNum (strict)"("Disabled"=w229, "Caption.Text"=w230) -> ()  [unwired: 2 in, 2 out]
                }
                frame 6 {
                  n138 = case shown="0, Default" w239 {
                    tunnel: [2 0 0 0] -> w240
                    tunnel: ["" ("Caption.Text") "mV/g" ("Caption.Text") "V/A" ("Caption.Text") "V/?" ("Caption.Text")] -> w241
                    frame 0, Default {
                    }
                    frame 1 {
                    }
                    frame 2 {
                    }
                    frame 3 {
                    }
                  }
                  n139 = property on="Scale Factor 7" class="DigNum (strict)"("Disabled"=w240, "Caption.Text"=w241) -> ()  [unwired: 2 in, 2 out]
                }
                frame 7 {
                  n140 = case shown="0, Default" w250 {
                    tunnel: [2 0 0 0] -> w251
                    tunnel: ["" ("Caption.Text") "mV/g" ("Caption.Text") "V/A" ("Caption.Text") "V/?" ("Caption.Text")] -> w252
                    frame 0, Default {
                    }
                    frame 1 {
                    }
                    frame 2 {
                    }
                    frame 3 {
                    }
                  }
                  n141 = property on="Scale Factor 8" class="DigNum (strict)"("Disabled"=w251, "Caption.Text"=w252) -> ()  [unwired: 2 in, 2 out]
                }
              }
            }
          }
          event "Ch 1 On/Off", "Ch 2 On/Off", "Ch 3 On/Off", "Ch 4 On/Off", "Analog Ouput On/Off", "Ch 5 On/Off", "Ch 6 On/Off", "Ch 7 On/Off", "Ch 8 On/Off": Value Change {
            # "Set the state to Idle"
            # "Update A/O LED"
            # "Update A/I LEDS"
            n142 = event-data() -> ()  [unwired: 1 in, 6 out]
            n143 = property on="Ch 5 On/Off" class="Bool (strict)"() -> ("Value"=→"Ch 5 LED":bool)  [unwired: 2 in, 2 out]
            n144 = property on="Ch 6 On/Off" class="Bool (strict)"() -> ("Value"=→"Ch 6 LED":bool)  [unwired: 2 in, 2 out]
            n145 = property on="Ch 7 On/Off" class="Bool (strict)"() -> ("Value"=→"Ch 7 LED":bool)  [unwired: 2 in, 2 out]
            n146 = property on="Ch 8 On/Off" class="Bool (strict)"() -> ("Value"=→"Ch 8 LED":bool)  [unwired: 2 in, 2 out]
            n147 = property on="Ch 1 On/Off" class="Bool (strict)"() -> ("Value"=→"Ch 1 LED":bool)  [unwired: 2 in, 2 out]
            n148 = property on="Ch 2 On/Off" class="Bool (strict)"() -> ("Value"=→"Ch 2 LED":bool)  [unwired: 2 in, 2 out]
            n149 = property on="Ch 3 On/Off" class="Bool (strict)"() -> ("Value"=→"Ch 3 LED":bool)  [unwired: 2 in, 2 out]
            n150 = property on="Ch 4 On/Off" class="Bool (strict)"() -> ("Value"=→"Ch 4 LED":bool)  [unwired: 2 in, 2 out]
            n151 = property on="Analog Ouput On/Off" class="Bool (strict)"() -> ("Value"=→"A/O LED":bool)  [unwired: 2 in, 2 out]
          }
          event "Exit": Value Change {
            # "Set the state to End"
            n152 = event-data() -> ()  [unwired: 1 in, 6 out]
          }
        }
      }
      frame "Execute" {
        w293 = -10.0  # Minimum Value (V) 8
        w294 = -10.0  # Minimum Value (V) 7
        w295 = -10.0  # Minimum Value (V) 6
        w296 = -10.0  # Minimum Value (V) 5
        w297 = 10.0  # Maximum Value (V) 8
        w298 = 10.0  # Maximum Value (V) 7
        w299 = 10.0  # Maximum Value (V) 6
        w300 = 10.0  # Maximum Value (V) 5
        w372 = 10123 items=["Finite Samples"=10178, "Continuous Samples"=10123] ("sample mode")
        w342 = -10.0  # Minimum Value (V) 4
        w340 = -10.0  # Minimum Value (V) 3
        w339 = -10.0  # Minimum Value (V) 2
        w341 = -10.0  # Minimum Value (V) 1
        w338 = 10.0  # Maximum Value (V) 4
        w337 = 10.0  # Maximum Value (V) 3
        w335 = 10.0  # Maximum Value (V) 2
        w336 = 10.0  # Maximum Value (V) 1
        # "Set the state to Idle"
        # "Update the Graph Labels and Time"
        # "Configure the Analog Input Channels and Start Acquisition"
        # "Configure the Analog Output Channel and Start Analog Output"
        # "Collect User Input and Build Cluster"
        # "Reset start, stop, and exit buttons"
        # "Perform data acquisition"
        n153 = Bundle("Ch 1 On/Off"="Ch 1 On/Off", "Ch 2 On/Off"="Ch 2 On/Off", "Ch 3 On/Off"="Ch 3 On/Off", "Ch 4 On/Off"="Ch 4 On/Off", "Ch 5 On/Off"="Ch 5 On/Off", "Ch 6 On/Off"="Ch 6 On/Off", "Ch 7 On/Off"="Ch 7 On/Off", "Ch 8 On/Off"="Ch 8 On/Off") -> (w351:T5)  [unwired: 1 in]
        n154 = Bundle("Physical Channel 1"="Physical Channel 1", "Physical Channel 2"="Physical Channel 2", "Physical Channel 3"="Physical Channel 3", "Physical Channel 4"="Physical Channel 4", "Physical Channel 5"="Physical Channel 5", "Physical Channel 6"="Physical Channel 6", "Physical Channel 7"="Physical Channel 7", "Physical Channel 8"="Physical Channel 8") -> (w343:T6)  [unwired: 1 in]
        n155 = Bundle("Minimum Value (V) 1"=w341, "Minimum Value (V) 2"=w339, "Minimum Value (V) 3"=w340, "Minimum Value (V) 4"=w342, "Minimum Value (V) 5"=w296, "Minimum Value (V) 6"=w295, "Minimum Value (V) 7"=w294, "Minimum Value (V) 8"=w293) -> (w345:T7)  [unwired: 1 in]
        n156 = control-ref of="Measurement"() -> (w364:refnum<vi>)
        n157 = control-ref of="Measurement 2"() -> (w365:refnum<vi>)
        n158 = control-ref of="Measurement 3"() -> (w366:refnum<vi>)
        n159 = control-ref of="Measurement 4"() -> (w367:refnum<vi>)
        n160 = control-ref of="Measurement 5"() -> (w312:refnum<vi>)
        n161 = control-ref of="Measurement 6"() -> (w311:refnum<vi>)
        n162 = control-ref of="Measurement 7"() -> (w310:refnum<vi>)
        n163 = control-ref of="Measurement 8"() -> (w309:refnum<vi>)
        n164 = Bundle("Scale Factor 8"="Scale Factor 8", "Scale Factor 7"="Scale Factor 7", "Scale Factor 6"="Scale Factor 6", "Scale Factor 5"="Scale Factor 5", "Scale Factor 4"="Scale Factor 4", "Scale Factor 3"="Scale Factor 3", "Scale Factor 2"="Scale Factor 2", "Scale Factor 1"="Scale Factor 1") -> (w363:T8)  [unwired: 1 in]
        n165 = Bundle("Maximum Value (V) 1"=w336, "Maximum Value (V) 2"=w335, "Maximum Value (V) 3"=w337, "Maximum Value (V) 4"=w338, "Maximum Value (V) 5"=w300, "Maximum Value (V) 6"=w299, "Maximum Value (V) 7"=w298, "Maximum Value (V) 8"=w297) -> (w344:T9)  [unwired: 1 in]
        n166 = Bundle("Channel Name 1"="Channel Name 1", "Channel Name 2"="Channel Name 2", "Channel Name 3"="Channel Name 3", "Channel Name 4"="Channel Name 4", "Channel Name 5"="Channel Name 5", "Channel Name 6"="Channel Name 6", "Channel Name 7"="Channel Name 7", "Channel Name 8"="Channel Name 8") -> (w346:T10)  [unwired: 1 in]
        n167 = Bundle("Channel Type 1"="Channel Type 1", "Channel Type 2"="Channel Type 2", "Channel Type 3"="Channel Type 3", "Channel Type 4"="Channel Type 4", "Channel Type 5"="Channel Type 5", "Channel Type 6"="Channel Type 6", "Channel Type 7"="Channel Type 7", "Channel Type 8"="Channel Type 8") -> (w362:T11)  [unwired: 1 in]
        n168 = Bundle("Measurement"=w364, "Measurement 2"=w365, "Measurement 3"=w366, "Measurement 4"=w367, "Measurement 5"=w312, "Measurement 6"=w311, "Measurement 7"=w310, "Measurement 8"=w309) -> (w368:T12)  [unwired: 1 in]
        n169 = Bundle(w368, w351, w346, w343, w344, w345, w362, w363) -> (w277:T13)  [unwired: 1 in]
        n170 = Unbundle(w277) -> (w377:T5)  [unwired: 7 out]
        n171 = invoke on="Start Acquisition" class="Bool (strict)" method="Reinit To Default"() -> ()  [unwired: 3 in, 3 out]
        n172 = call "8CHDAQ - Create Channels.vi"("Channel Data"=w277) -> ("error out"=w278:errorcluster, "task out"=w279:refnum<k21>)  [unwired: 9 in]
        n173 = property on="Start Acquisition" class="Bool (strict)"("Disabled"=u8 2) -> ()  [unwired: 2 in, 2 out]
        n174 = property on="Stop Acquisition" class="Bool (strict)"("Disabled"=u8 0) -> ()  [unwired: 2 in, 2 out]
        n175 = property on="Exit" class="Bool (strict)"("Disabled"=u8 2) -> ()  [unwired: 2 in, 2 out]
        n176 = Unbundle(w377) -> ("Ch 1 On/Off"=w378:bool, "Ch 2 On/Off"=w379:bool, "Ch 3 On/Off"=w380:bool, "Ch 4 On/Off"=w381:bool, "Ch 5 On/Off"=w284:bool, "Ch 6 On/Off"=w283:bool, "Ch 7 On/Off"=w282:bool, "Ch 8 On/Off"=w281:bool)
        n177 = Multiply(x="Rate", y=50.0) -> (x*y=w375:dbl)
        n178 = Build Array(w378, w379, w380, w381, w284, w283, w282, w281) -> (w382:bool[])
        n179 = call-poly <vilib>:"DAQmx Timing.vi"("task/channels in"=w279, "sample mode"=w372, "samples per channel"=w375, "rate"="Rate", "error in"=w278) -> ("task out"=w373:refnum<k21>, "error out"=w374:errorcluster)  [unwired: 9 in]
        n180 = case shown="True" "Analog Ouput On/Off" {
          tunnel: [_ w568] -> w370
          tunnel: [_ w567] -> w369
          tunnel: "Channel Name" -> [_ w564]
          tunnel: "Physical Channel" -> [_ w563]
          tunnel: "Desired Frequency" -> [_ w562]
          tunnel: "Waveform Type" -> [_ w561]
          tunnel: "Amplitude" -> [_ w560]
          tunnel: "Cycles per Buffer" -> [_ w559]
          tunnel: [_ w558] -> w376
          frame False {
          }
          frame True {
            n181 = call "4CHDAQ - Configure Analog Output.vi"("Cycles per Buffer"=w559, "Channel Name"=w564, "Amplitude"=w560, "Desired Frequency"=w562, "Waveform Type"=w561, "Physical Channels"=w563) -> ("error out"=w566:errorcluster, "Resulting Frequency"=w558:dbl, "task out"=w565:refnum<k21>)  [unwired: 3 in]
            n182 = call <vilib>:"DAQmx Start Task.vi"("task/channels in"=w565, "error in"=w566) -> ("task out"=w568:refnum<k21>, "error out"=w567:errorcluster)  [unwired: 12 in]
          }
        }
        "Resulting Frequency" <- w376
        n183 = call <vilib>:"DAQmx Start Task.vi"("task/channels in"=w373, "error in"=w374) -> ("task out"=w322:refnum<k21>, "error out"=w321:errorcluster)  [unwired: 12 in]
        n184 = property class="DAQmx Timing"(reference=w322, error in=w321) -> (reference out=w320:refnum<k21>, error out=w319:errorcluster, "SampClk.Rate"=w276:dbl)
        "Sampling Freq" <- w276
        n185 = Multiply(x="Graph Time", y=w276) -> (x*y=w280:dbl)
        n186 = call "8CHDAQ - Update Plot Ledgend and Scale.vi"("Max"=w280, "Channel Data"=w277) -> ()  [unwired: 10 in]
        n187 = flat-sequence {
          tunnel: w369 -> [w405]
          tunnel: w370 -> [w404]
          tunnel: w319 -> [w402]
          tunnel: w320 -> [w401]
          tunnel: w382 -> [w399]
          tunnel: [w398] -> w384
          tunnel: "Analog Ouput On/Off" -> [w390]
          tunnel: w277 -> [w389]
          tunnel: w276 -> [w386]
          tunnel: w277 -> [w549]
          tunnel: w384 -> [w550]
          tunnel: w276 -> [w548]
          frame #0 {
            w400 = T14 3 items=["no dialog", "OK message", "continue or stop message", "OK message + warnings", "continue/stop + warnings"] ("type of dialog (OK msg:1)")
            # "Stop Acquisition and Display and Errors"
            n188 = Divide(x=w386, y="Refresh Rate") -> (x/y=w388:dbl)
            n189 = Round To Nearest(number=w388) -> (nearest integer value=w387:dbl)
            n190 = while {
              tunnel: [w464] -> w395
              tunnel: w401 -> [w467]
              tunnel: w402 -> [w466]
              tunnel: [w465] -> w396
              tunnel: w387 -> [w461]
              tunnel: w404 -> [w460]
              tunnel: w405 -> [w459]
              tunnel: [w460] -> w392
              tunnel: [w459] -> w391
              tunnel: w399 -> [w456]
              shift-right: [w449] -> w398
              shift-left: dbl[][] [] -> [w454]
              tunnel: w389 -> [w450]
              stop <- w452 stop-if-true
              w462 = 10.0  # timeout
              # "Display Data on Respective Graphs"
              # "Scale Data and Build Data Array"
              # "Read Data from Analog Input Channels"
              # "Stop on Error or \"Stop Acquisition\" button"
              n191 = call-poly <vilib>:"DAQmx Read.vi"("task/channels in"=w467, "number of samples per channel"=w461, "timeout"=w462, "error in"=w466) -> ("task out"=w465:refnum<k21>, "data"=w451:dbl[][], "error out"=w464:errorcluster)  [unwired: 9 in]
              n192 = Decimal String To Number(string="Input Signal Measurement Channel") -> (number=w436:i32)  [unwired: 2 in, 1 out]
              n193 = call "8CHDAQ - Scale Data.vi"("Array Input"=w451, "Channel Data"=w450) -> ("Array Output"=w435:dbl[][])  [unwired: 9 in]
              n194 = Unbundle By Name(w464) -> ("status"=w463:bool)
              n195 = Index Array(array=w435, index (row)=w436) -> (element=w434:dbl[])  [unwired: 1 in]
              n196 = Transpose 2D Array(2D array=w435) -> (transposed array=w453:dbl[][])
              n197 = Bundle By Name("Y"=w434) -> (w433:waveform(dbl))  [unwired: 1 in]
              n198 = for {
                N: 8 -> [_]
                tunnel: w456 -> [w486] mode=indexing
                shift-right: [w478] -> _
                shift-left: 0 ("index") -> [w483]
                tunnel: w435 -> [w484]
                tunnel: w433 -> [w482]
                tunnel: [w481] -> w416 mode=indexing
                tunnel: [w480] -> w415 mode=indexing
                tunnel: [w479] -> w414 mode=indexing
                i -> [w485]
                n199 = case shown="True" w486 {
                  tunnel: w485 -> [_ w499]
                  tunnel: w484 -> [_ w498]
                  tunnel: w483 -> [w490 w496]
                  tunnel: [w490 w497] -> w478
                  tunnel: w482 -> [_ w494]
                  tunnel: [cluster{"f0":dbl, "df":dbl, "magnitude":dbl[]} {"f0"=0.0, "df"=0.0, "magnitude"=[]} ("magnitude") w493] -> w481
                  tunnel: [cluster{"f0":dbl, "df":dbl, "phase":dbl[]} {"f0"=0.0, "df"=0.0, "phase"=[]} ("phase") w492] -> w480
                  tunnel: [cluster{"f0":dbl, "df":dbl, "coherence":dbl[]} {"f0"=0.0, "df"=0.0, "coherence"=[]} ("coherence") w491] -> w479
                  frame False {
                  }
                  frame True {
                    n200 = Index Array(array=w498, index (row)=w496) -> (element=w495:dbl[])  [unwired: 1 in]
                    n201 = case shown="1" w499 {
                      tunnel: w495 -> [w504 w510 w516 w522 w524 w534 w540 w542]
                      tunnel: w494 -> [w503 w509 w512 w521 w525 w533 w539 w543]
                      tunnel: [w502 w508 w515 w520 w528 w532 w538 w546] -> w493
                      tunnel: [w501 w507 w514 w519 w527 w531 w537 w545] -> w492
                      tunnel: [w500 w506 w513 w518 w526 w530 w536 w544] -> w491
                      frame 0, Default {
                        n202 = Bundle By Name("Y"=w504) -> (w505:waveform(dbl))  [unwired: 1 in]
                        n203 = call-poly <vilib>:"Frequency Response Function (Mag-Phase).vi"("time signal X"=w503, "time signal Y"=w505) -> ("magnitude"=w502:cluster{"f0":dbl, "df":dbl, "magnitude":dbl[]}, "phase"=w501:cluster{"f0":dbl, "df":dbl, "phase":dbl[]}, "coherence"=w500:cluster{"f0":dbl, "df":dbl, "coherence":dbl[]})  [unwired: 8 in, 3 out]
                        "Measurement" <- w504
                      }
                      frame 1 {
                        n204 = Bundle By Name("Y"=w510) -> (w511:waveform(dbl))  [unwired: 1 in]
                        n205 = call-poly <vilib>:"Frequency Response Function (Mag-Phase).vi"("time signal X"=w509, "time signal Y"=w511) -> ("magnitude"=w508:cluster{"f0":dbl, "df":dbl, "magnitude":dbl[]}, "phase"=w507:cluster{"f0":dbl, "df":dbl, "phase":dbl[]}, "coherence"=w506:cluster{"f0":dbl, "df":dbl, "coherence":dbl[]})  [unwired: 8 in, 3 out]
                        "Measurement 2" <- w510
                      }
                      frame 2 {
                        n206 = Bundle By Name("Y"=w516) -> (w517:waveform(dbl))  [unwired: 1 in]
                        n207 = call-poly <vilib>:"Frequency Response Function (Mag-Phase).vi"("time signal X"=w512, "time signal Y"=w517) -> ("magnitude"=w515:cluster{"f0":dbl, "df":dbl, "magnitude":dbl[]}, "phase"=w514:cluster{"f0":dbl, "df":dbl, "phase":dbl[]}, "coherence"=w513:cluster{"f0":dbl, "df":dbl, "coherence":dbl[]})  [unwired: 8 in, 3 out]
                        "Measurement 3" <- w516
                      }
                      frame 3 {
                        n208 = Bundle By Name("Y"=w522) -> (w523:waveform(dbl))  [unwired: 1 in]
                        n209 = call-poly <vilib>:"Frequency Response Function (Mag-Phase).vi"("time signal X"=w521, "time signal Y"=w523) -> ("magnitude"=w520:cluster{"f0":dbl, "df":dbl, "magnitude":dbl[]}, "phase"=w519:cluster{"f0":dbl, "df":dbl, "phase":dbl[]}, "coherence"=w518:cluster{"f0":dbl, "df":dbl, "coherence":dbl[]})  [unwired: 8 in, 3 out]
                        "Measurement 4" <- w522
                      }
                      frame 4 {
                        n210 = Bundle By Name("Y"=w524) -> (w529:waveform(dbl))  [unwired: 1 in]
                        n211 = call-poly <vilib>:"Frequency Response Function (Mag-Phase).vi"("time signal X"=w525, "time signal Y"=w529) -> ("magnitude"=w528:cluster{"f0":dbl, "df":dbl, "magnitude":dbl[]}, "phase"=w527:cluster{"f0":dbl, "df":dbl, "phase":dbl[]}, "coherence"=w526:cluster{"f0":dbl, "df":dbl, "coherence":dbl[]})  [unwired: 8 in, 3 out]
                        "Measurement 5" <- w524
                      }
                      frame 5 {
                        n212 = Bundle By Name("Y"=w534) -> (w535:waveform(dbl))  [unwired: 1 in]
                        n213 = call-poly <vilib>:"Frequency Response Function (Mag-Phase).vi"("time signal X"=w533, "time signal Y"=w535) -> ("magnitude"=w532:cluster{"f0":dbl, "df":dbl, "magnitude":dbl[]}, "phase"=w531:cluster{"f0":dbl, "df":dbl, "phase":dbl[]}, "coherence"=w530:cluster{"f0":dbl, "df":dbl, "coherence":dbl[]})  [unwired: 8 in, 3 out]
                        "Measurement 6" <- w534
                      }
                      frame 6 {
                        n214 = Bundle By Name("Y"=w540) -> (w541:waveform(dbl))  [unwired: 1 in]
                        n215 = call-poly <vilib>:"Frequency Response Function (Mag-Phase).vi"("time signal X"=w539, "time signal Y"=w541) -> ("magnitude"=w538:cluster{"f0":dbl, "df":dbl, "magnitude":dbl[]}, "phase"=w537:cluster{"f0":dbl, "df":dbl, "phase":dbl[]}, "coherence"=w536:cluster{"f0":dbl, "df":dbl, "coherence":dbl[]})  [unwired: 8 in, 3 out]
                        "Measurement 7" <- w540
                      }
                      frame 7 {
                        n216 = Bundle By Name("Y"=w542) -> (w547:waveform(dbl))  [unwired: 1 in]
                        n217 = call-poly <vilib>:"Frequency Response Function (Mag-Phase).vi"("time signal X"=w543, "time signal Y"=w547) -> ("magnitude"=w546:cluster{"f0":dbl, "df":dbl, "magnitude":dbl[]}, "phase"=w545:cluster{"f0":dbl, "df":dbl, "phase":dbl[]}, "coherence"=w544:cluster{"f0":dbl, "df":dbl, "coherence":dbl[]})  [unwired: 8 in, 3 out]
                        "Measurement 8" <- w542
                      }
                    }
                    n218 = Increment(x=w496) -> (x+1=w497:i32)
                  }
                }
              }
              "FRF Coherence" <- w414
              "FRF Phase" <- w415
              "FRF Magnitude" <- w416
              n219 = Build Array (concatenate)(w454, w453) -> (w449:dbl[][])
              n220 = Or(x=w463, y="Stop Acquisition") -> (x .or. y?=w452:bool)
              n221 = Index Array(array=w435, index (row) #1=0 ("index"), index (row) #2=1 ("index"), index (row) #3=2 ("index"), index (row) #4=3 ("index"), index (row) #5=4 ("index"), index (row) #6=5 ("index"), index (row) #7=6 ("index"), index (row) #8=7 ("index")) -> (element #1=w417:dbl[], element #2=w418:dbl[], element #3=w419:dbl[], element #4=w420:dbl[], element #5=w421:dbl[], element #6=w422:dbl[], element #7=w423:dbl[], element #8=w424:dbl[])  [unwired: 8 in]
              n222 = Bundle By Name("Y"=w417) -> (w432:waveform(dbl))  [unwired: 1 in]
              n223 = Bundle By Name("Y"=w418) -> (w431:waveform(dbl))  [unwired: 1 in]
              n224 = Bundle By Name("Y"=w419) -> (w430:waveform(dbl))  [unwired: 1 in]
              n225 = Bundle By Name("Y"=w420) -> (w429:waveform(dbl))  [unwired: 1 in]
              n226 = Bundle By Name("Y"=w421) -> (w428:waveform(dbl))  [unwired: 1 in]
              n227 = Bundle By Name("Y"=w422) -> (w427:waveform(dbl))  [unwired: 1 in]
              n228 = Bundle By Name("Y"=w423) -> (w426:waveform(dbl))  [unwired: 1 in]
              n229 = Bundle By Name("Y"=w424) -> (w425:waveform(dbl))  [unwired: 1 in]
              n230 = Merge Signals(w432, w431, w430, w429, w428, w427, w426, w425) -> (w448:dynamicdata)
              n231 = xnode "Spectral Measurements"("Signals"=w448) -> ("FFT - (RMS)"=→"FFT Magnitude":dynamicdata, "Phase"=→"FFT Phase":dynamicdata)  [unwired: 1 in, 1 out]
            }
            n232 = case shown="True" w390 {
              tunnel: w392 -> [_ w409]
              tunnel: w391 -> [_ w408]
              frame False {
              }
              frame True {
                w412 = T14 3 items=["no dialog", "OK message", "continue or stop message", "OK message + warnings", "continue/stop + warnings"] ("type of dialog (OK msg:1)")
                # "Stop Analog Output and Display and Errors"
                n233 = call "4CHDAQ - Clear AO Channel.vi"("error in"=w408, "task/channels in"=w409) -> ("error out"=w406:errorcluster, "task out"=w407:refnum<k21>)  [unwired: 8 in]
                n234 = call <vilib>:"DAQmx Stop Task.vi"("task/channels in"=w407, "error in"=w406) -> ("task out"=w411:refnum<k21>, "error out"=w410:errorcluster)  [unwired: 12 in]
                n235 = call <vilib>:"DAQmx Clear Task.vi"("task in"=w411, "error in"=w410) -> ("error out"=w413:errorcluster)  [unwired: 13 in]
                n236 = call <vilib>:"Simple Error Handler.vi"("type of dialog (OK msg:1)"=w412, "error in (no error)"=w413) -> ()  [unwired: 3 in, 5 out]
              }
            }
            n237 = call <vilib>:"DAQmx Stop Task.vi"("task/channels in"=w396, "error in"=w395) -> ("task out"=w394:refnum<k21>, "error out"=w393:errorcluster)  [unwired: 12 in]
            n238 = call <vilib>:"DAQmx Clear Task.vi"("task in"=w394, "error in"=w393) -> ("error out"=w403:errorcluster)  [unwired: 13 in]
            n239 = call <vilib>:"Simple Error Handler.vi"("type of dialog (OK msg:1)"=w400, "error in (no error)"=w403) -> ()  [unwired: 3 in, 5 out]
          }
          frame #1 {
            # "Prompt User to Save Data File"
            n240 = Two Button Dialog(message="Save Data File?", 1:"No" ("F button name (\"Cancel\")"), 2:"Yes" ("T button name (\"OK\")")) -> (T button?=w551:bool)
            n241 = case shown="True" w551 {
              tunnel: w550 -> [_ w556]
              tunnel: w549 -> [_ w557]
              tunnel: w548 -> [_ w555]
              frame False {
              }
              frame True {
                # "Save the Data File"
                n242 = call "8CHDAQ - Save Data File.vi"("Array"=w556, "Sampling Rate"=w555, "Channel Data"=w557) -> ()  [unwired: 9 in]
              }
            }
          }
        }
      }
      frame "End" {
      }
    }
    n243 = Equal?(x=w3, y=enum16{"Initialize", "Idle", "Execute", "End"}."End") -> (x = y?=w5:bool)
  }
